vi "BURST mode U2000A.vi"() -> ()   [LabVIEW 2025]
uses:
  <vilib>/Instr/_visa.llb/VISA Open Access Mode.ctl
  e2d0d99d-9bb7-4129-8f6c-a154af6e61e9.vi
  <vilib>/Utility/error.llb/Trim Whitespace One-Sided.vi
  <instrlib>/Agilent U2000 Series/Agilent U2000 Series.lvlib
panel:
  in  "Wait to Fetch":u32=3000
  out "error out":errorcluster
  out "Measurement":dbl
  out "Command":string
  out "read buffer":string
  in  "error in (no error)":errorcluster
  in  "VISA resource name":refnum<visa-resource-name>
  in  "FETCH only":bool
  # "FALSE - Full setting\nTRUE - Fetch only"
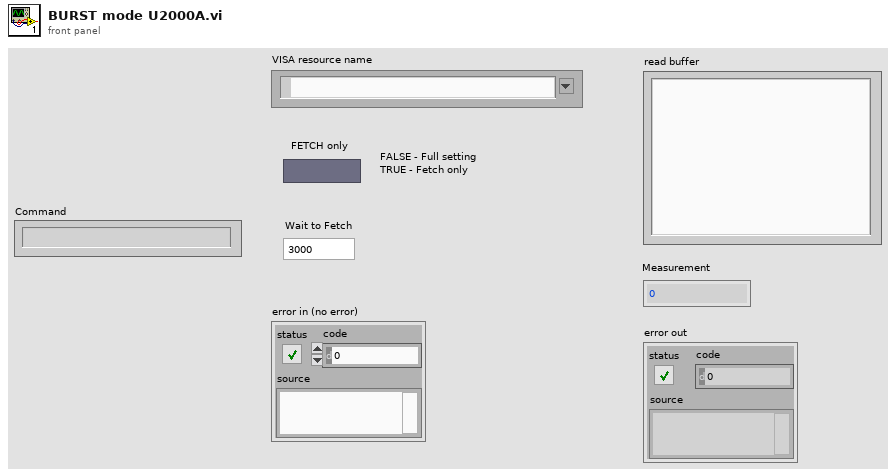
[diagram p1: front panel]
types:
  T1 = typedef "VISA Open Access Mode.ctl" = u32
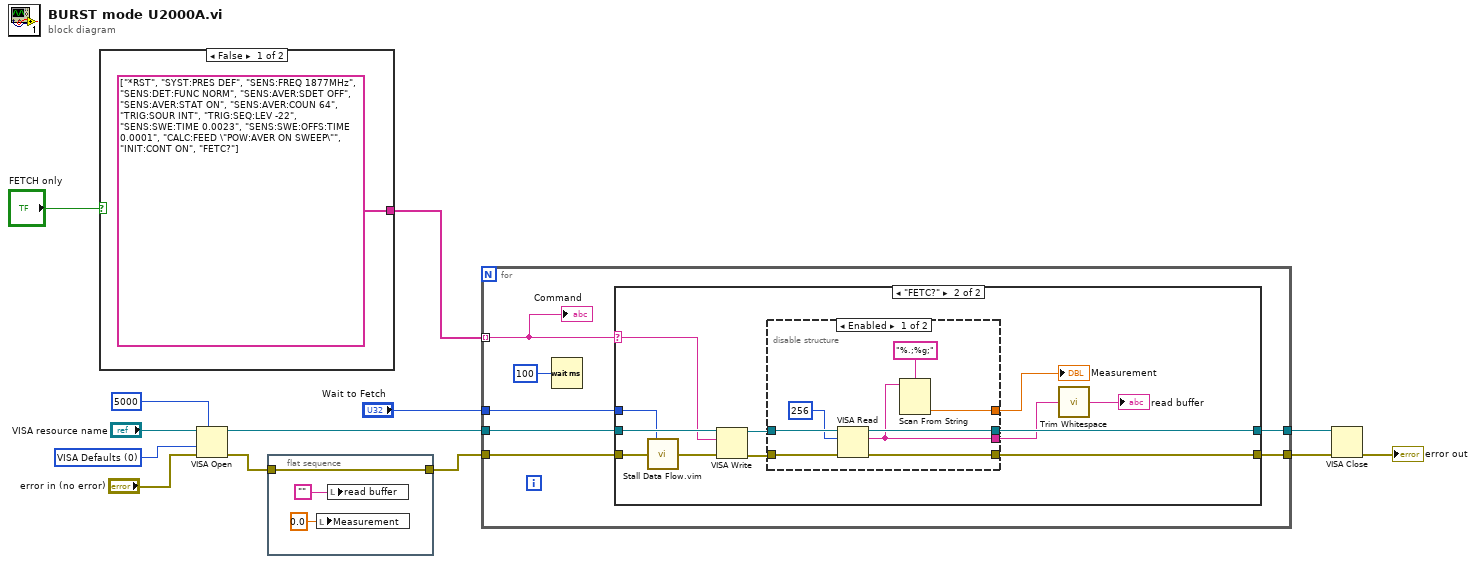
[diagram p0: block diagram]
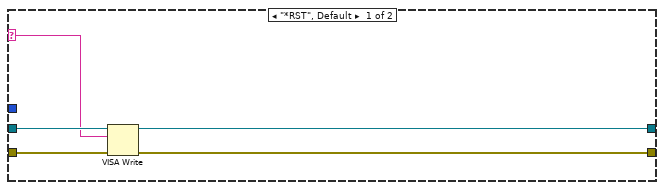
[diagram p2: hidden frame]
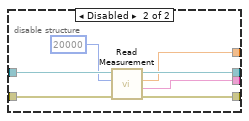
[diagram p3: hidden frame]
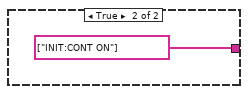
[diagram p4: hidden frame]
diagram:
  w12 = T1 0 items=["VISA Defaults"=0, "Exclusive Lock"=1, "Load Configured Settings"=4] ("Access Mode")
  n1 = case shown="False" "FETCH only" {
    tunnel: [string[] ["*RST", "SYST:PRES DEF", "SENS:FREQ 1877MHz", "SENS:DET:FUNC NORM", "SENS:AVER:SDET OFF", "SENS:AVER:STAT ON", "SENS:AVER:COUN 64", "TRIG:SOUR INT", "TRIG:SEQ:LEV -22", "SENS:SWE:TIME 0.0023", "SENS:SWE:OFFS:TIME 0.0001", "CALC:FEED \"POW:AVER ON SWEEP\"", "INIT:CONT ON", "FETC?"] string[] ["INIT:CONT ON"]] -> w4
    frame False {
    }
    frame True {
    }
  }
  n2 = VISA Open(timeout (0)=u32 5000 ("VISA Open timeout (0)"), access mode=w12, error in (no error)="error in (no error)", VISA resource name="VISA resource name") -> (VISA resource name=w8:refnum<visa-resource-name>, error out=w3:errorcluster)  [unwired: 1 in]
  n3 = flat-sequence {
    tunnel: w3 -> [w16]
    tunnel: [w16] -> w2
    frame #0 {
      n4 = local write "Measurement"(0.0 ("Measurement")) -> ()
      n5 = local write "read buffer"("") -> ()
    }
  }
  n6 = for {
    tunnel: w4 -> [w25] mode=indexing
    tunnel: [w24] -> w7
    tunnel: [w23] -> w6
    tunnel: w2 -> [w22]
    tunnel: w8 -> [w21]
    tunnel: "Wait to Fetch" -> [w19]
    n7 = Wait (ms)(milliseconds to wait=u32 100) -> ()  [unwired: 1 out]
    n8 = case shown="\"FETC?\"" w25 {
      selector: w25 -> [w26 w34]
      tunnel: [w27 w42] -> w23
      tunnel: [w28 w41] -> w24
      tunnel: w22 -> [w30 w39]
      tunnel: w21 -> [w29 w36]
      tunnel: w19 -> [_ w31]
      frame "*RST", Default {
        n9 = VISA Write(VISA resource name=w29, write buffer=w26, error in (no error)=w30) -> (VISA resource name out=w27:refnum<visa-resource-name>, error out=w28:errorcluster)  [unwired: 1 out]
      }
      frame "FETC?" {
        n10 = call "Stall Data Flow.vim"("value in"=w39, "milliseconds to wait"=w31) -> ("value out"=w38:errorcluster)  [unwired: 1 out]
        n11 = VISA Write(VISA resource name=w36, write buffer=w34, error in (no error)=w38) -> (VISA resource name out=w35:refnum<visa-resource-name>, error out=w37:errorcluster)  [unwired: 1 out]
        n12 = disable-structure shown="Enabled" {
          disable-tunnel: w35 -> [w50 w57]
          disable-tunnel: [w49 w56] -> w42
          disable-tunnel: [w44 w53] -> w32
          disable-tunnel: [w48 w54] -> w41
          disable-tunnel: w37 -> [w46 w55]
          disable-tunnel: [w43 w52] -> w40
          frame Enabled {
            n13 = VISA Read(VISA resource name=w50, byte count=u32 256, error in (no error)=w46) -> (VISA resource name out=w49:refnum<visa-resource-name>, read buffer=w44:string, error out=w48:errorcluster)  [unwired: 1 out]
            n14 = Scan From String(format string="%.;%g;", input string=w44) -> (output 1=w43:dbl)  [unwired: 2 in, 4 out]
          }
          frame Disabled {
            n15 = call <instrlib>:"Read Measurement.vi"("error in (no error)"=w55, "Timeout (10000 ms)"=u32 20000 ("milliseconds to wait"), "VISA resource name"=w57) -> ("error out"=w54:errorcluster, "read buffer"=w53:string, "Measurement"=w52:dbl, "VISA resource name out"=w56:refnum<visa-resource-name>)  [unwired: 5 in]
          }
        }
        "Measurement" <- w40
        n16 = call <vilib>:"Trim Whitespace.vi"("string"=w32) -> ("trimmed string"=→"read buffer":string)  [unwired: 1 in]
      }
    }
    "Command" <- w25
  }
  n17 = VISA Close(VISA resource name=w6, error in (no error)=w7) -> (error out=→"error out":errorcluster)
